vi "Task2_ex2.vi"() -> ()   [LabVIEW 2024]
doc: "Use this template to build a producer/consumer design pattern. Use this template when you need to execute a process, such as data analysis, when a data source, such as a triggered acquisition, produces data at an uneven rate and you need to execute the process when the data becomes available."
uses:
  <vilib>/DAQmx/read.llb/DAQmx Read (Analog 2D DBL NChan NSamp).vi
  <vilib>/DAQmx/miscellaneous.llb/DAQmx Fill In Error Info.vi
panel:
  out "data":dbl[][](graph)
  in  "stop 2":bool caption="stop"
  in  "stop":bool
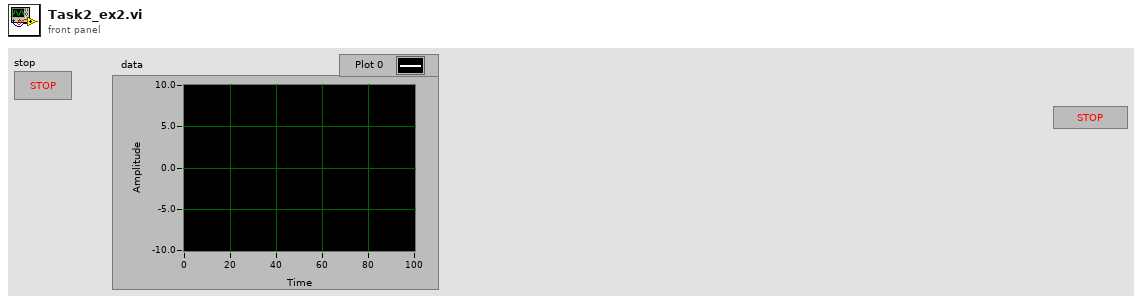
[diagram p1: front panel]
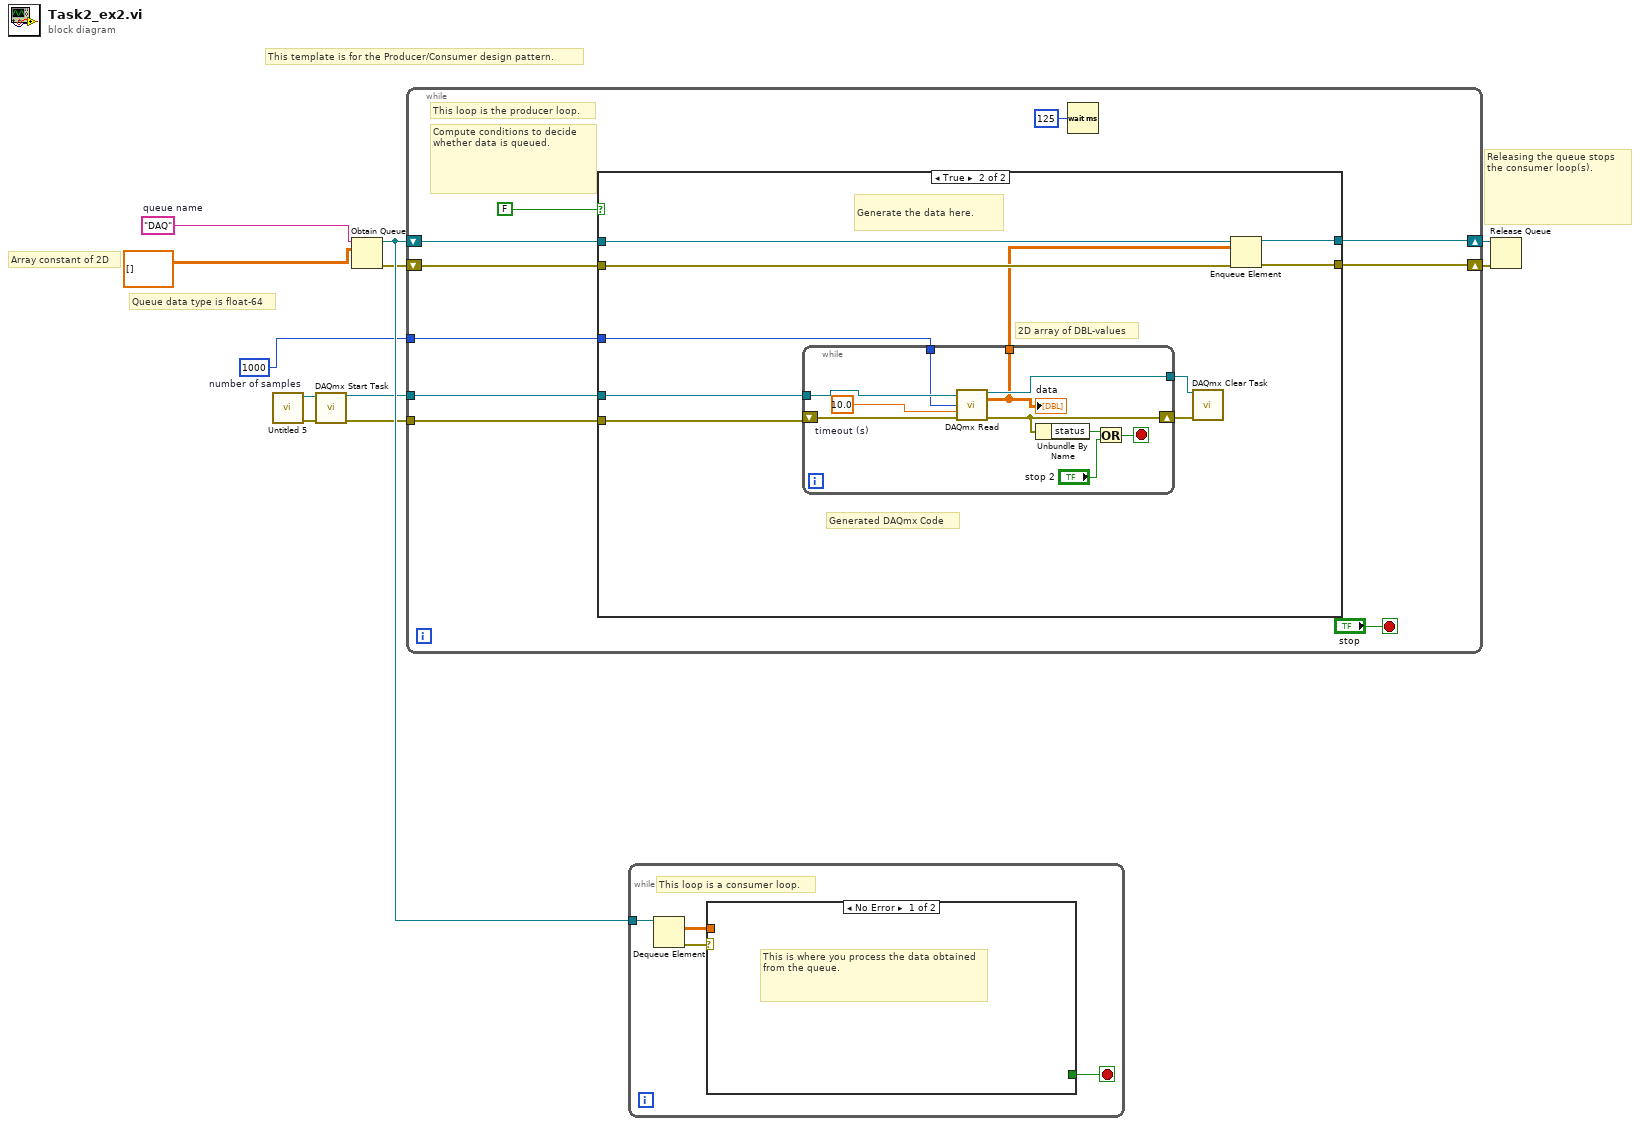
[diagram p0: block diagram]
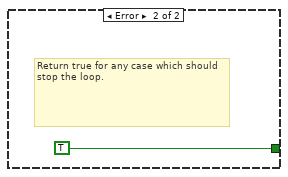
[diagram p2: hidden frame]
diagram:
  w6 = 1000  # number of samples
  w2 = "DAQ"  # queue name
  # "Queue data type is float-64"
  # "Array constant of 2D"
  # "Releasing the queue stops the consumer loop(s)."
  # "This template is for the Producer/Consumer design pattern."
  n1 = call "Untitled 5.vi"() -> ("error out"=w4:errorcluster, "task out"=w5:refnum<k21>)  [unwired: 10 in]
  n2 = call <vilib>:"DAQmx Start Task.vi"("task/channels in"=w5, "error in"=w4) -> ("task out"=w7:refnum<k21>, "error out"=w3:errorcluster)  [unwired: 12 in]
  n3 = Obtain Queue(name (unnamed)=w2, element data type=dbl[][] []) -> (queue out=w11:refnum<queue>, error out=w10:errorcluster)  [unwired: 3 in, 1 out]
  n4 = while {
    shift-right: [w17] -> w8
    shift-left: w10 -> [w18]
    shift-right: [w19] -> w9
    shift-left: w11 -> [w20]
    tunnel: w7 -> [w14]
    tunnel: w6 -> [w13]
    tunnel: w3 -> [w12]
    stop <- "stop" stop-if-true
    # "Compute conditions to decide whether data is queued."
    # "This loop is the producer loop."
    n5 = case shown="True" FALSE ("Case Constant\n(See Context Help)") {
      tunnel: w20 -> [w23 w33]
      tunnel: [w23 w32] -> w19
      tunnel: w18 -> [w22 w31]
      tunnel: [w22 w30] -> w17
      tunnel: w14 -> [_ w27]
      tunnel: w13 -> [_ w26]
      tunnel: w12 -> [_ w25]
      frame False {
      }
      frame True {
        # "2D array of DBL-values"
        # "Generated DAQmx Code"
        # "Generate the data here."
        n6 = while {
          tunnel: [w42] -> w29
          shift-right: [w40] -> w28
          shift-left: w25 -> [w43]
          tunnel: w27 -> [w36]
          tunnel: w26 -> [w35]
          tunnel: [w34] -> w24
          stop <- w39 stop-if-true
          w37 = 10.0  # timeout (s)
          n7 = call-poly <vilib>:"DAQmx Read.vi"("task/channels in"=w36, "number of samples per channel"=w35, "timeout"=w37, "error in"=w43) -> ("task out"=w42:refnum<k21>, "data"=w34:dbl[][], "error out"=w40:errorcluster)  [unwired: 9 in]
          "data" <- w34
          n8 = Unbundle By Name(w40) -> ("status"=w41:bool)
          n9 = Or(x=w41, y="stop 2") -> (x .or. y?=w39:bool)
        }
        n10 = call <vilib>:"DAQmx Clear Task.vi"("task in"=w29, "error in"=w28) -> ()  [unwired: 13 in, 1 out]
        n11 = Enqueue Element(queue=w33, element=w24, error in (no error)=w31) -> (queue out=w32:refnum<queue>, error out=w30:errorcluster)  [unwired: 1 in, 1 out]
      }
    }
    n12 = Wait (ms)(milliseconds to wait=u32 125) -> ()  [unwired: 1 out]
  }
  n13 = while {
    tunnel: w11 -> [w47]
    stop <- w44 stop-if-true
    # "This loop is a consumer loop."
    n14 = Dequeue Element(queue=w47) -> (element=w45:dbl[][], error out=w46:errorcluster)  [unwired: 2 in, 2 out]
    n15 = case shown="No Error" w46 {
      tunnel: w45 -> [_ _]
      tunnel: [_ TRUE] -> w44
      frame No Error {
        # "This is where you process the data obtained from the queue."
      }
      frame Error {
        # "Return true for any case which should stop the loop."
      }
    }
  }
  n16 = Release Queue(queue=w9, error in (no error)=w8) -> ()  [unwired: 1 in, 3 out]
